vi "pistof1.vi"() -> ()   [LabVIEW 2019]
uses:
  <vilib>/Instr/_visa.llb/VISA Configure Serial Port (Instr).vi
panel:
  out "hPa":string
  out "dB":string
  out "temp":string
  in  "stop":bool
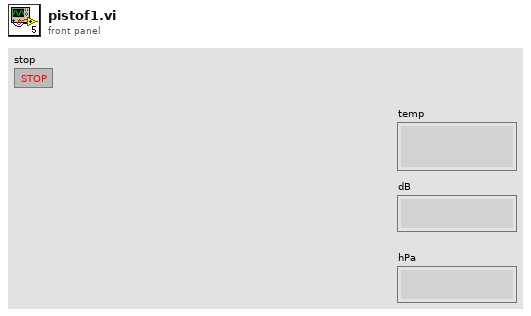
[diagram p1: front panel]
types:
  T1 = cluster{"baud rate":u32, "data bits":u16, "parity":enum16{"None", "Odd", "Even", "Mark", "Space"}, "stop bits":u16, "flow control":u16}
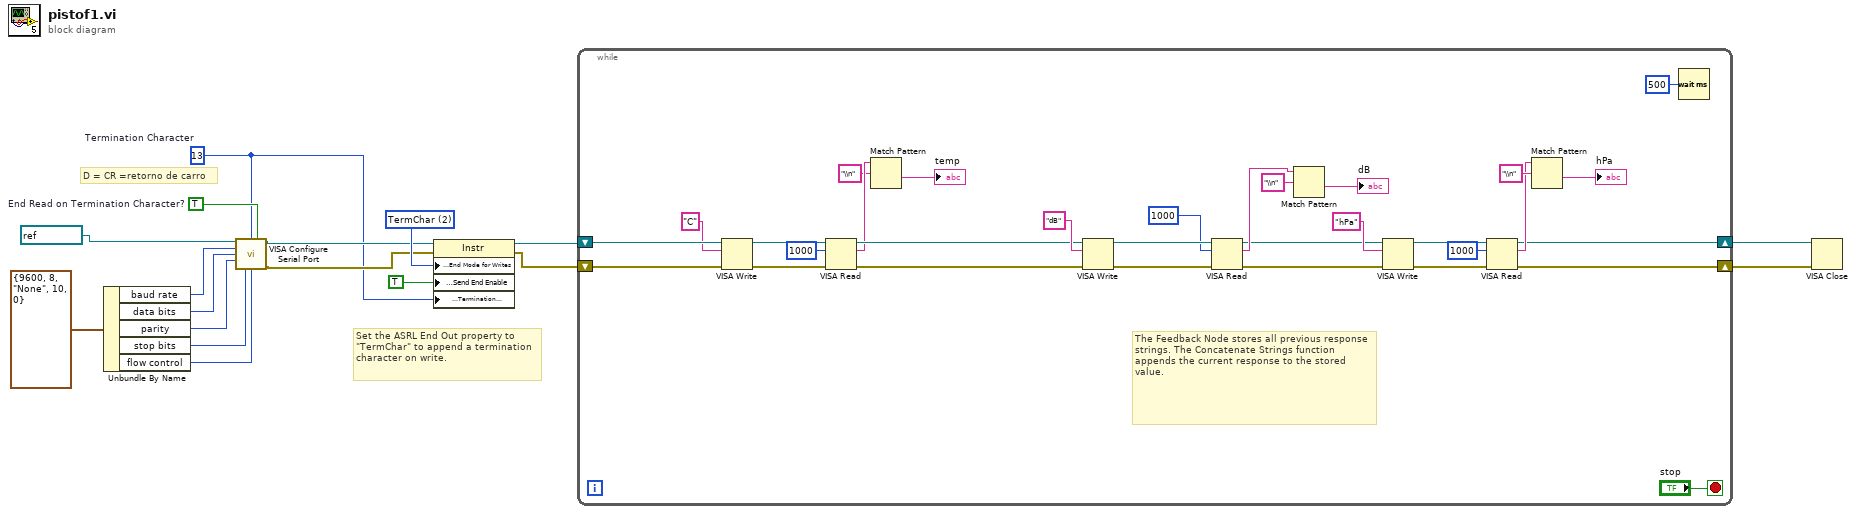
[diagram p0: block diagram]
diagram:
  w6 = u16 2 items=["None", "LastBit", "TermChar", "Break"] ("Serial Settings:Serial End Mode for Writes")
  w1 = u8 13  # Termination Character
  w12 = TRUE  # End Read on Termination Character?
  # "Set the ASRL End Out property to \"TermChar\" to append a termination character on write."
  # "D = CR =retorno de carro"
  n1 = Unbundle By Name(T1 {"baud rate"=9600, "data bits"=8, "parity"=enum."None", "stop bits"=10, "flow control"=0} ("Serial Settings")) -> ("baud rate"=w14:u32, "data bits"=w15:u16, "parity"=w16:enum16{"None", "Odd", "Even", "Mark", "Space"}, "stop bits"=w17:u16, "flow control"=w9:u16)
  n2 = call-poly "VISA Configure Serial Port"("VISA resource name"=refnum<visa-resource-name> "COM3", "termination char\n(0xA = '\\n' = LF)"=w1, "Enable Termination\nChar (T)"=w12, "baud rate (9600)"=w14, "data bits (8)"=w15, "parity (0:none)"=w16, "stop bits (10: 1 bit)"=w17, "flow control (0:none)"=w9) -> ("VISA resource name out"=w5:refnum<visa-resource-name>, "error out"=w4:errorcluster)  [unwired: 2 in, 4 out]
  n3 = property class="Instr"(reference=w5, error in=w4, "Serial Settings:End Mode for Writes"=w6, "Message Based Settings:Send End Enable"=TRUE, "Message Based Settings:Termination Character"=w1) -> (reference out=w3:refnum<visa-resource-name>, error out=w2:errorcluster)
  n4 = while {
    shift-right: [w18] -> w11
    shift-left: w2 -> [w48]
    shift-right: [w19] -> w10
    shift-left: w3 -> [w40]
    stop <- "stop" stop-if-true
    # "The Feedback Node stores all previous response strings. The Concatenate Strings function appends the current response to the stored value."
    n5 = VISA Write(VISA resource name=w40, write buffer="C", error in (no error)=w48) -> (VISA resource name out=w37:refnum<visa-resource-name>, error out=w41:errorcluster)  [unwired: 1 out]
    n6 = VISA Read(VISA resource name=w37, byte count=u32 1000, error in (no error)=w41) -> (VISA resource name out=w36:refnum<visa-resource-name>, read buffer=w34:string, error out=w38:errorcluster)  [unwired: 1 out]
    n7 = Match Pattern(string=w34, regular expression="\\n") -> (after substring=→"temp":string)  [unwired: 1 in, 3 out]
    n8 = VISA Write(VISA resource name=w36, write buffer="dB" ("Command"), error in (no error)=w38) -> (VISA resource name out=w47:refnum<visa-resource-name>, error out=w46:errorcluster)  [unwired: 1 out]
    n9 = VISA Read(VISA resource name=w47, byte count=u32 1000 ("Read Count"), error in (no error)=w46) -> (VISA resource name out=w21:refnum<visa-resource-name>, read buffer=w30:string, error out=w20:errorcluster)  [unwired: 1 out]
    n10 = Match Pattern(string=w30, regular expression="\\n") -> (after substring=→"dB":string)  [unwired: 1 in, 3 out]
    n11 = VISA Write(VISA resource name=w21, write buffer="hPa", error in (no error)=w20) -> (VISA resource name out=w24:refnum<visa-resource-name>, error out=w22:errorcluster)  [unwired: 1 out]
    n12 = VISA Read(VISA resource name=w24, byte count=u32 1000, error in (no error)=w22) -> (VISA resource name out=w19:refnum<visa-resource-name>, read buffer=w26:string, error out=w18:errorcluster)  [unwired: 1 out]
    n13 = Match Pattern(string=w26, regular expression="\\n") -> (after substring=→"hPa":string)  [unwired: 1 in, 3 out]
    n14 = Wait (ms)(milliseconds to wait=u32 500) -> ()  [unwired: 1 out]
  }
  n15 = VISA Close(VISA resource name=w10, error in (no error)=w11) -> ()  [unwired: 1 out]
